vi "String_ENA3G Parameters.vi"(8 "error in (no error)":errorcluster, 11 "String":string="Spectrum from 1.0E+5 Hz to 1.0E+6 Hz, Bandwidth 25.00 Hz, 201 points, Power -20.00 dB") -> (0 "error out":errorcluster, 1 "MeasConfig":T1={"Tiempo (sec)"=10.0, "Campo X (T)"=0.025, "Campo Y (T)"=10.0, "Campo Z (T)"=0.025, "Temperatura (K)"=0.025, "Start Frequency (Hz)"=100000.0, "Stop Frequency (Hz)"=1000000.0, "IF Bandwidth"=25.0, "Sweep time(s)"=25.0, "Meas Points"=201, "Power Level (0.0)"=-40.0} {"Campo Z (T)" format="%^.2e"; "Campo Y (T)" format="%^.2e"; "Sweep time(s)" format="%^.2g"; "Temperatura (K)" format="%^.2e"; "Campo X (T)" format="%^.2e"; "Tiempo (sec)" format="%^.2g"; "Start Frequency (Hz)" format="%^.2e"; "IF Bandwidth" format="%^.2e"; "Power Level (0.0)" format="%^.2g"})   [LabVIEW 2017]
uses:
  RohdeSchwarz ZNB MeasConfig.ctl
panel:
  out "# Points (2..1601)":u16=201
  out "IF Bandwidth (Hz)":dbl=25.0 format="%.1f"
  out "Stop Frequency (Hz)":dbl=1000000.0 format="%^.2e"
  out "Start Frequency (Hz)":dbl=100000.0 format="%^.2e"
  out "Power Level (dB)":dbl=-20.0 format="%.2f"
  # "Spectrum from 1.0E+5 Hz to 1.0E+6 Hz, Bandwidth 25.00 Hz, 201 points, Power -20.00 dB"
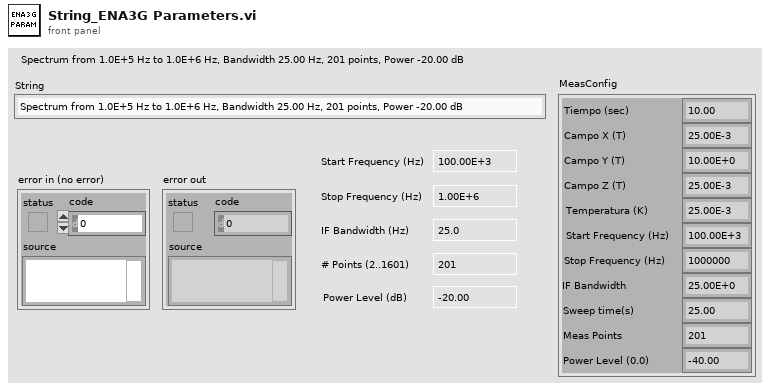
[diagram p1: front panel]
types:
  T1 = typedef "RohdeSchwarz ZNB MeasConfig.ctl" = cluster{"Tiempo (sec)":dbl, "Campo X (T)":dbl, "Campo Y (T)":dbl, "Campo Z (T)":dbl, "Temperatura (K)":dbl, "Start Frequency (Hz)":dbl, "Stop Frequency (Hz)":dbl, "IF Bandwidth":dbl, "Sweep time(s)":dbl, "Meas Points":i32, "Power Level (0.0)":dbl}
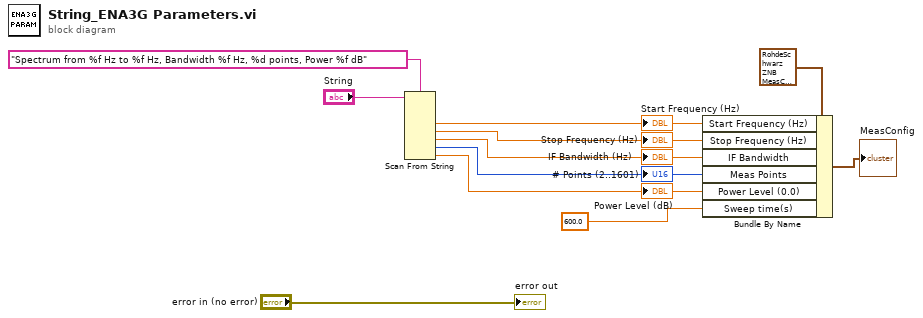
[diagram p0: block diagram]
diagram:
  n1 = Scan From String(format string="Spectrum from %f Hz to %f Hz, Bandwidth %f Hz, %d points, Power %f dB", input string="String") -> (output 1=w7:dbl, output 2=w6:dbl, output 3=w3:dbl, output 4=w5:u16, output 5=w4:dbl)  [unwired: 7 in, 3 out]
  "# Points (2..1601)" <- w5
  "IF Bandwidth (Hz)" <- w3
  "Stop Frequency (Hz)" <- w6
  "Start Frequency (Hz)" <- w7
  "Power Level (dB)" <- w4
  n2 = Bundle By Name(cluster=T1 {"Tiempo (sec)"=10.0, "Campo X (T)"=0.025, "Campo Y (T)"=10.0, "Campo Z (T)"=0.025, "Temperatura (K)"=0.025, "Start Frequency (Hz)"=100000.0, "Stop Frequency (Hz)"=1000000.0, "IF Bandwidth"=25.0, "Sweep time(s)"=25.0, "Meas Points"=201, "Power Level (0.0)"=-40.0} ("MeasConfig"), "Start Frequency (Hz)"=w7, "Stop Frequency (Hz)"=w6, "IF Bandwidth"=w3, "Meas Points"=w5, "Power Level (0.0)"=w4, "Sweep time(s)"=600.0) -> (→"MeasConfig":T1)
  "error out" <- "error in (no error)"
